vi "Write Command.vi"(8 "error in (no error)":errorcluster, 10 "Command":T1, 11 "DriveData in":refnum<class "DriveData.lvclass">) -> (0 "error out":errorcluster, 3 "DriveData out":refnum<class "DriveData.lvclass">)   [LabVIEW 2017, in "DriveData.lvclass"]
uses:
  DriveData.lvclass
  Command.ctl
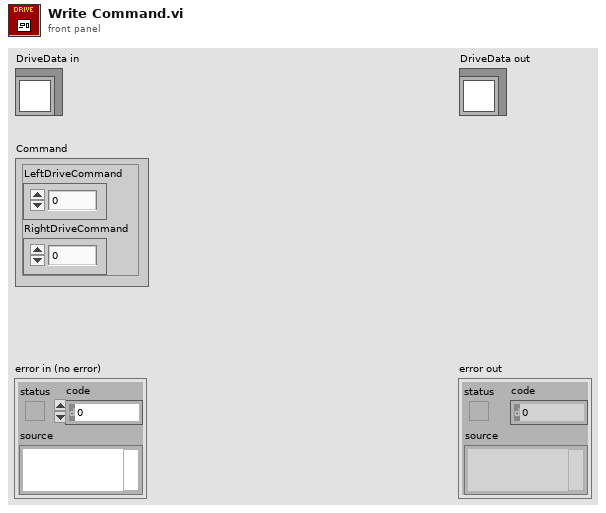
[diagram p1: front panel]
types:
  T1 = typedef "DriveData.lvclass/Command.ctl" = cluster{"LeftDriveCommand":dbl, "RightDriveCommand":dbl}
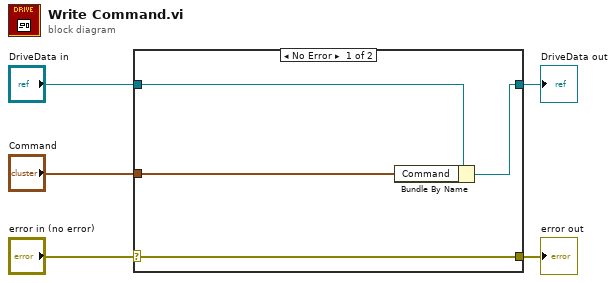
[diagram p0: block diagram]
diagram:
  n1 = case shown="No Error" "error in (no error)" {
    selector: "error in (no error)" -> [w9 w10]
    tunnel: [w9 w10] -> w4
    tunnel: [w7 w11] -> w2
    tunnel: "DriveData in" -> [w8 w11]
    tunnel: "Command" -> [w6 _]
    frame No Error {
      n2 = Bundle By Name(cluster=w8, "Command"=w6) -> (w7:refnum<class "DriveData.lvclass">)
    }
    frame Error {
    }
  }
  "error out" <- w4
  "DriveData out" <- w2
